vi "selfConfigRead.vi"(0 "RefDesType":string, 5 "error in":errorcluster) -> (12 "Control refDes concat":string[](array[string]), 14 "DAQ Node Array":string[](array[string]), 15 "DAQ Node Count":i32, 16 "refDes":string, 17 "IPaddr":string, 18 "Control refDes array":string[][](array[string]), 19 "error out":errorcluster)   [LabVIEW 2024]
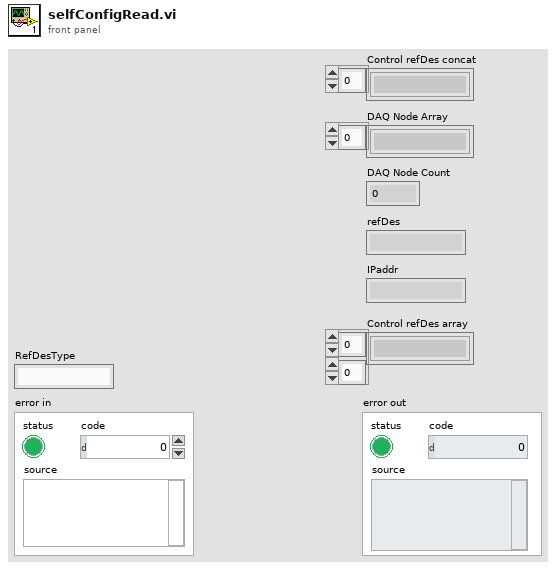
[diagram p1: front panel]
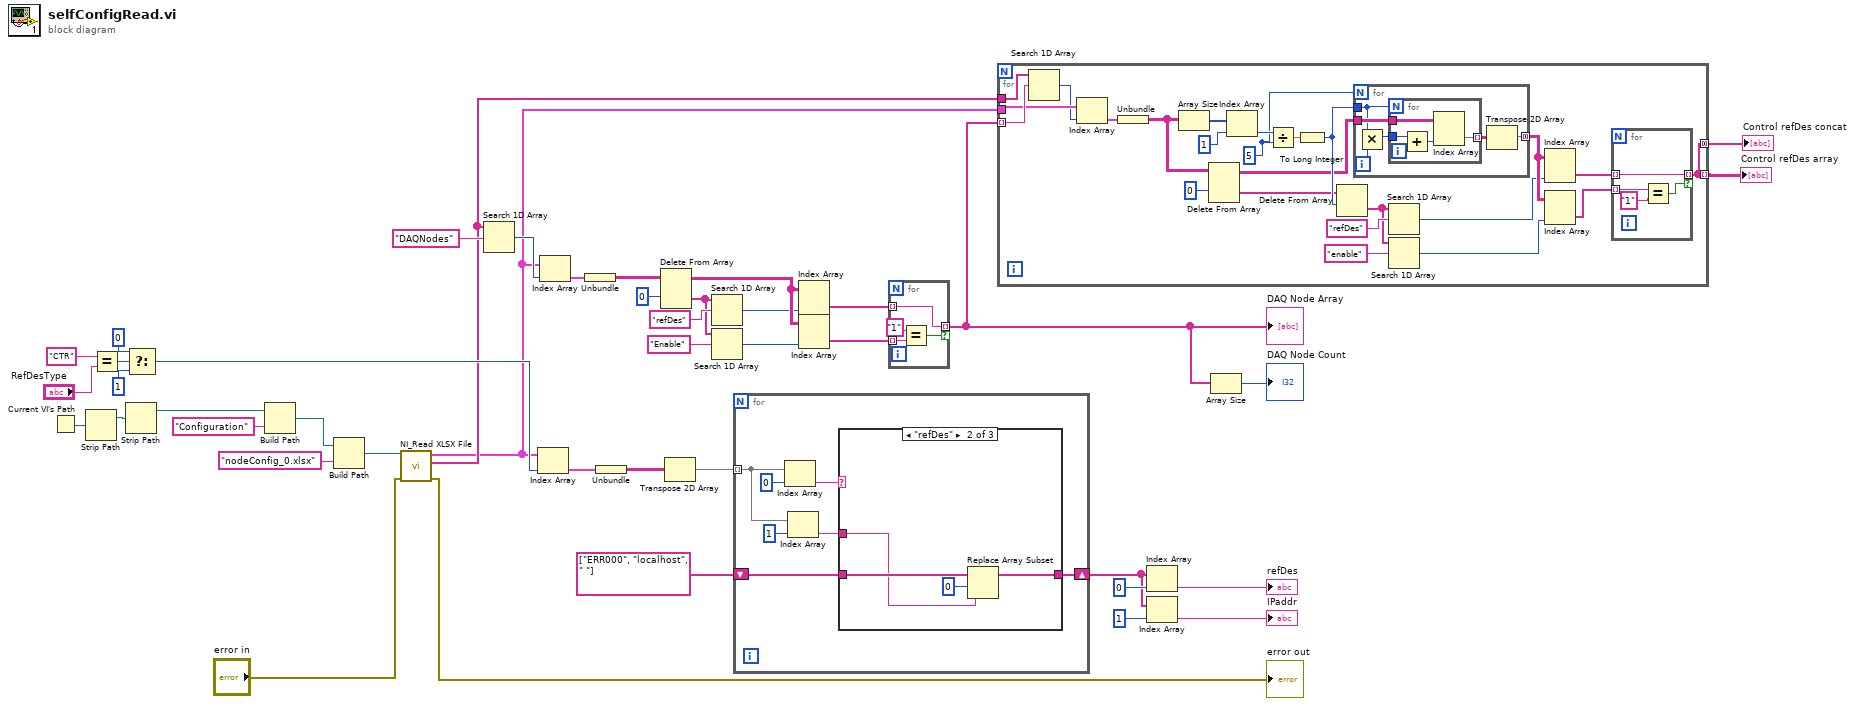
[diagram p0: block diagram]
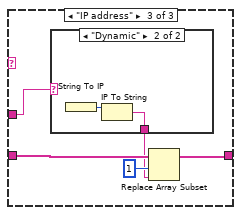
[diagram p3: hidden frame]
diagram:
  n1 = Current VI's Path() -> (path=w41:path)
  n2 = Strip Path(path=w41) -> (stripped path=w33:path)  [unwired: 1 out]
  n3 = Equal?(x="CTR", y="RefDesType") -> (x = y?=w29:bool)
  n4 = Strip Path(path=w33) -> (stripped path=w32:path)  [unwired: 1 out]
  n5 = Select(t=0, s=w29, f=1) -> (s? t:f=w26:i32)
  n6 = Build Path(base path=w32, name or relative path="Configuration") -> (appended path=w34:path)
  n7 = Build Path(base path=w34, name or relative path="nodeConfig_0.xlsx") -> (appended path=w42:path)
  n8 = call "NI_Read XLSX File.vi"("error in"="error in", "XLSX File"=w42) -> ("error out"=→"error out":errorcluster, "Sheet Names"=w4:string[], "Sheet Data"=w3:cluster{"Array":string[][]}[])  [unwired: 7 in]
  n9 = Search 1D Array(1D array=w4, element="DAQNodes") -> (index of element=w18:i32)  [unwired: 1 in]
  n10 = Index Array(array=w3, index=w26) -> (element=w25:cluster{"Array":string[][]})
  n11 = Index Array(array=w3, index=w18) -> (element=w17:cluster{"Array":string[][]})
  n12 = Unbundle(w17) -> ("Array"=w13:string[][])
  n13 = Unbundle(w25) -> ("Array"=w24:string[][])
  n14 = Delete From Array(array=w13, index (row)=0) -> (deleted portion=w12:string[], array with subset deleted=w11:string[][])  [unwired: 2 in]
  n15 = Transpose 2D Array(2D array=w24) -> (transposed array=w23:string[][])
  n16 = Search 1D Array(1D array=w12, element="refDes") -> (index of element=w9:i32)  [unwired: 1 in]
  n17 = Search 1D Array(1D array=w12, element="Enable") -> (index of element=w10:i32)  [unwired: 1 in]
  n18 = for {
    tunnel: w23 -> [w48] mode=indexing
    shift-right: [w45] -> w21
    shift-left: string[] ["ERR000", "localhost", " "] -> [w46]
    n19 = Index Array(array=w48, index=0) -> (element=w47:string)
    n20 = Index Array(array=w48, index=1) -> (element=w44:string)
    n21 = case shown="\"refDes\"" w47 {
      tunnel: w46 -> [w51 w55 w59]
      tunnel: [w51 w54 w58] -> w45
      tunnel: w44 -> [_ w52 w57]
      frame Default {
      }
      frame "refDes" {
        n22 = Replace Array Subset(array=w55, new element=w52, index=0) -> (w54:string[])
      }
      frame "IP address" {
        n23 = case shown="\"Dynamic\"" w57 {
          selector: w57 -> [w61 _]
          tunnel: [w61 w62] -> w56
          frame Default {
          }
          frame "Dynamic" {
            n24 = String To IP() -> (0:w63:u32)  [unwired: 1 in]
            n25 = IP To String(2:w63) -> (0:w62:string)  [unwired: 1 in]
          }
        }
        n26 = Replace Array Subset(array=w59, new element=w56, index=1) -> (w58:string[])
      }
    }
  }
  n27 = Index Array(array=w11, index (col)=w9) -> (element=w8:string[])  [unwired: 1 in]
  n28 = Index Array(array=w11, index (col)=w10) -> (element=w7:string[])  [unwired: 1 in]
  n29 = for {
    tunnel: w8 -> [w65] mode=indexing
    tunnel: w7 -> [w67] mode=indexing
    tunnel: [w65] -> w5 mode=indexing if=w64
    n30 = Equal?(x="1", y=w67) -> (x = y?=w64:bool)
  }
  "DAQ Node Array" <- w5
  n31 = for {
    tunnel: w5 -> [w91] mode=indexing
    tunnel: w4 -> [w90]
    tunnel: w3 -> [w89]
    tunnel: [w68] -> w2 mode=indexing
    tunnel: [w68] -> w1 mode=concatenating
    w74 = 5 ("y")
    n32 = Search 1D Array(1D array=w90, element=w91) -> (index of element=w88:i32)  [unwired: 1 in]
    n33 = Index Array(array=w89, index=w88) -> (element=w87:cluster{"Array":string[][]})
    n34 = Unbundle(w87) -> ("Array"=w71:string[][])
    n35 = Array Size(array=w71) -> (size(s)=w75:i32[])
    n36 = Delete From Array(array=w71, index (row)=0) -> (deleted portion=w81:string[], array with subset deleted=w82:string[][])  [unwired: 2 in]
    n37 = Index Array(array=w75, index=1) -> (element=w76:i32)
    n38 = Divide(x=w76, y=w74) -> (x/y=w77:dbl)
    n39 = To Long Integer(number=w77) -> (32bit integer=w83:i32)
    n40 = Delete From Array(array=w81, length=w83) -> (deleted portion=w78:string[])  [unwired: 1 in, 1 out]
    n41 = for {
      N: w74 -> [_]
      tunnel: w82 -> [w101]
      tunnel: w83 -> [w99]
      tunnel: [w96] -> w85 mode=concatenating
      i -> [w100]
      n42 = Multiply(x=w99, y=w100) -> (x*y=w98:i32)
      n43 = for {
        N: w99 -> [_]
        tunnel: w101 -> [w106]
        tunnel: w98 -> [w104]
        tunnel: [w102] -> w97 mode=indexing
        i -> [w105]
        n44 = Add(x=w104, y=w105) -> (x+y=w103:i32)
        n45 = Index Array(array=w106, index (col)=w103) -> (element=w102:string[])  [unwired: 1 in]
      }
      n46 = Transpose 2D Array(2D array=w97) -> (transposed array=w96:string[][])
    }
    n47 = Search 1D Array(1D array=w78, element="refDes") -> (index of element=w84:i32)  [unwired: 1 in]
    n48 = Search 1D Array(1D array=w78, element="enable") -> (index of element=w86:i32)  [unwired: 1 in]
    n49 = Index Array(array=w85, index (col)=w84) -> (element=w70:string[])  [unwired: 1 in]
    n50 = Index Array(array=w85, index (col)=w86) -> (element=w69:string[])  [unwired: 1 in]
    n51 = for {
      tunnel: [w95] -> w68 mode=indexing if=w92
      tunnel: w70 -> [w95] mode=indexing
      tunnel: w69 -> [w94] mode=indexing
      n52 = Equal?(x=w94, y="1") -> (x = y?=w92:bool)
    }
  }
  "Control refDes array" <- w2
  "Control refDes concat" <- w1
  n53 = Index Array(array=w21, index=0) -> (element=→"refDes":string)
  n54 = Index Array(array=w21, index=1) -> (element=→"IPaddr":string)
  n55 = Array Size(array=w5) -> (size(s)=→"DAQ Node Count":i32)
